vi "Create Incremental Numeric File Name (SubVI).vi"(10 "folder":path, 11 "file extension":string) -> (3 "String":string)   [LabVIEW 2020, in "FileIO.lvlib"]
uses:
  FileIO.lvlib
panel:
  out "file names":string[](array[string])
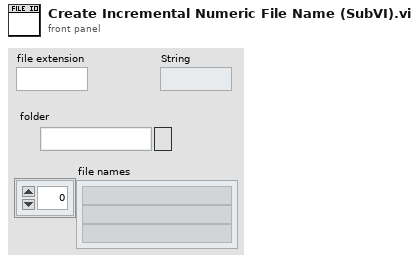
[diagram p1: front panel]
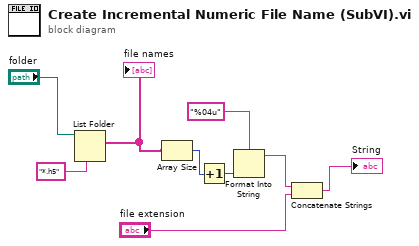
[diagram p0: block diagram]
diagram:
  n1 = List Folder(path="folder", pattern="*.h5") -> (filenames=w2:string[])  [unwired: 2 in, 3 out]
  "file names" <- w2
  n2 = Array Size(array=w2) -> (size(s)=w4:i32)
  n3 = Increment(x=w4) -> (x+1=w1:i32)
  n4 = Format Into String(format string="%04u", w1) -> (resulting string=w3:string)  [unwired: 2 in, 1 out]
  n5 = Concatenate Strings(w3, "file extension") -> (→"String":string)
